vi "open motors.vi"() -> ()   [LabVIEW 2019]
uses:
  <vilib>/Rock Robotics/WPI/ThirdParty/Phoenix-LabVIEW/Motor Controller/Controls/CTRE_Phoenix_MotorControl_TalonFXMotorControllerConfigurables.ctl
  <vilib>/Rock Robotics/WPI/ThirdParty/Phoenix-LabVIEW/Motor Controller/Controls/CTRE_Phoenix_MotorControl_BaseConfigurables.ctl
  <vilib>/Rock Robotics/WPI/ThirdParty/Phoenix-LabVIEW/Motor Controller/Controls/CTRE_Phoenix_MotorControl_VelocityMeasurementPeriod.ctl
  <vilib>/Rock Robotics/WPI/ThirdParty/Phoenix-LabVIEW/Motor Controller/Controls/CTRE_Phoenix_MotorControl_SlotStructure.ctl
  <vilib>/Rock Robotics/WPI/ThirdParty/Phoenix-LabVIEW/Motor Controller/Controls/CTRE_Phoenix_MotorControl_FilterStruct.ctl
  <vilib>/Rock Robotics/WPI/ThirdParty/Phoenix-LabVIEW/Motor Controller/Controls/CTRE_Phoenix_MotorControl_RemoteSourceType.ctl
  <vilib>/Rock Robotics/WPI/ThirdParty/Phoenix-LabVIEW/Controls/CTRE_Phoenix_CustomParamConfiguration.ctl
  <vilib>/Rock Robotics/WPI/ThirdParty/Phoenix-LabVIEW/Motor Controller/Controls/CTRE_Phoenix_MotorControl_FeedbackDevice_TalonFX.ctl
  <vilib>/Rock Robotics/WPI/ThirdParty/Phoenix-LabVIEW/Motor Controller/Controls/CTRE_Phoenix_MotorControl_LimitSwitchNormal.ctl
  <vilib>/Rock Robotics/WPI/ThirdParty/Phoenix-LabVIEW/Motor Controller/Controls/CTRE_Phoenix_MotorControl_LimitSwitchSource_Local.ctl
  <vilib>/Rock Robotics/WPI/ThirdParty/Phoenix-LabVIEW/Motor Controller/Controls/CTRE_Phoenix_MotorControl_SupplyCurrentLimitConfiguration.ctl
  <vilib>/Rock Robotics/WPI/ThirdParty/Phoenix-LabVIEW/Motor Controller/Controls/CTRE_Phoenix_MotorControl_StatorCurrentLimitConfiguration.ctl
  <vilib>/Rock Robotics/WPI/ThirdParty/Phoenix-LabVIEW/Motor Controller/Controls/CTRE_Phoenix_MotorControl_MotorCommutation_TalonFX.ctl
  <vilib>/Rock Robotics/WPI/ThirdParty/Phoenix-LabVIEW/CANCoder/Controls/CTRE_Phoenix_CANcoder_AbsoluteSensorRange.ctl
  <vilib>/Rock Robotics/WPI/ThirdParty/Phoenix-LabVIEW/CANCoder/Controls/CTRE_Phoenix_CANcoder_SensorInitializationStrategy.ctl
  <vilib>/Rock Robotics/WPI/ThirdParty/Phoenix-LabVIEW/Motor Controller/Controls/CTRE_Phoenix_MotorControl_StatusFrameEnhanced.ctl
  <vilib>/Rock Robotics/WPI/ThirdParty/Phoenix-LabVIEW/Motor Controller/Controls/CTRE_Phoenix_MotorControl_EnhancedMotorControllerConfigurables.ctl
  <vilib>/Rock Robotics/WPI/ThirdParty/Phoenix-LabVIEW/Motor Controller/Controls/CTRE_Phoenix_MotorControl_FeedbackDevice.ctl
  <vilib>/Rock Robotics/WPI/ThirdParty/Phoenix-LabVIEW/Motor Controller/Controls/CTRE_Phoenix_MotorControl_SensorTermFeedbackDevice_Enhanced.ctl
  <vilib>/Rock Robotics/WPI/RobotDrive/WPI_RobotDriveOpen4MotorWithExistingMotors.vi
panel:
  in  "Talon FX Configurables":T1={"Base Configurables"={"openLoopRamp"=0.0, "closedLoopRamp"=0.0, "peakOutputForward"=1.0, "peakOutputReverse"=-1.0, "nominalOutputForward"=0.0, "nominalOutputReverse"=0.0, "neutralDeadband"=0.04, "voltageCompSaturation"=0.0, "voltageMeasurementFilter"=32, "velocityMeasurementPeriod"=100, "velocityMeasurementWindow"=64, "forwardSoftLimitThreshold"=0, "reverseSoftLimitThreshold"=0, "forwardSoftLimitEnable"=FALSE, "reverseSoftLimitEnable"=FALSE, "slot0"={"P"=0.0, "I"=0.0, "D"=0.0, "F"=0.0, "integralZone"=0.0, "allowableClosedLoopError"=0, "maxIntegralAccumulator"=0.0, "closedLoopPeakOutput"=1.0, "closedLoopPeriod"=1}, "slot1"={"P"=0.0, "I"=0.0, "D"=0.0, "F"=0.0, "integralZone"=0.0, "allowableClosedLoopError"=0, "maxIntegralAccumulator"=0.0, "closedLoopPeakOutput"=1.0, "closedLoopPeriod"=1}, "slot2"={"P"=0.0, "I"=0.0, "D"=0.0, "F"=0.0, "integralZone"=0.0, "allowableClosedLoopError"=0, "maxIntegralAccumulator"=0.0, "closedLoopPeakOutput"=1.0, "closedLoopPeriod"=1}, "slot3"={"P"=0.0, "I"=0.0, "D"=0.0, "F"=0.0, "integralZone"=0.0, "allowableClosedLoopError"=0, "maxIntegralAccumulator"=0.0, "closedLoopPeakOutput"=1.0, "closedLoopPeriod"=1}, "auxPIDPolarity"=FALSE, "remoteFilter0"={"remoteSensorDeviceID"=0, "remoteSensorSource"=enum."Off"}, "remoteFilter1"={"remoteSensorDeviceID"=0, "remoteSensorSource"=enum."Off"}, "motionCruiseVelocity"=0, "motionAcceleration"=0, "motionProfileTrajectoryPeriod"=0, "feedbackNotContinuous"=FALSE, "remoteSensorClosedLoopDisableNeutralOnLOS"=FALSE, "clearPositionOnLimitF"=FALSE, "clearPositionOnLimitR"=FALSE, "clearPositionOnQuadIdx"=FALSE, "limitSwitchDisableNeutralOnLOS"=FALSE, "softLimitDisableNeutralOnLOS"=FALSE, "pulseWidthPeriod_EdgesPerRot"=1, "pulseWidthPeriod_FilterWindowSz"=1, "customParam"={"customParam0"=0, "customParam1"=0}, "trajectoryInterpolationEnable"=TRUE}, "primaryPID"={"selectedFeedbackCoefficient"=1.0, "selectedFeedbackSensor"=1}, "auxiliaryPID"={"selectedFeedbackCoefficient"=1.0, "selectedFeedbackSensor"=1}, "forwardLimitSwitchNormal"=enum."Normally Open", "reverseLimitSwitchNormal"=enum."Normally Open", "forwardLimitSwitchDeviceID"=0, "reverseLimitSwitchDeviceID"=0, "forwardLimitSwitchSource"=enum."Feedback Connector", "reverseLimitSwitchSource"=enum."Feedback Connector", "sum0Term"=1, "sum1Term"=1, "diff0Term"=1, "diff1Term"=1, "Supply Current Limit Configuration"={"Enable?"=FALSE, "Current Limit"=0.0, "Threshold Current"=0.0, "Threshold Time"=0.0}, "Stator Current Limit Configuration"={"Enable?"=FALSE, "Current Limit"=0.0, "Threshold Current"=0.0, "Threshold Time"=0.0}, "Motor Commutation"=enum."Trapezoidal", "Absolute Sensor Range"=enum."Unsigned [0 to 360)", "Integrated Sensor Offset (Degrees)"=0.0, "Sensor Initialization Strategy"=enum."Boot To Zero"} {"diff1Term" items=["Integrated Sensor"=1, "Sensor Sum (S0 + S1)"=9, "Sensor Difference (D0 - D1)"=10, "Remote Source 0"=11, "Remote Source 1"=12, "None"=14, "Software Emulated"=15]; "diff0Term" items=["Integrated Sensor"=1, "Sensor Sum (S0 + S1)"=9, "Sensor Difference (D0 - D1)"=10, "Remote Source 0"=11, "Remote Source 1"=12, "None"=14, "Software Emulated"=15]; "sum1Term" items=["Integrated Sensor"=1, "Sensor Sum (S0 + S1)"=9, "Sensor Difference (D0 - D1)"=10, "Remote Source 0"=11, "Remote Source 1"=12, "None"=14, "Software Emulated"=15]; "sum0Term" items=["Integrated Sensor"=1, "Sensor Sum (S0 + S1)"=9, "Sensor Difference (D0 - D1)"=10, "Remote Source 0"=11, "Remote Source 1"=12, "None"=14, "Software Emulated"=15]; "auxiliaryPID"."selectedFeedbackSensor" items=["Integrated Sensor"=1, "Sensor Sum (S0 + S1)"=9, "Sensor Difference (D0 - D1)"=10, "Remote Source 0"=11, "Remote Source 1"=12, "None"=14, "Software Emulated"=15]; "primaryPID"."selectedFeedbackSensor" items=["Integrated Sensor"=1, "Sensor Sum (S0 + S1)"=9, "Sensor Difference (D0 - D1)"=10, "Remote Source 0"=11, "Remote Source 1"=12, "None"=14, "Software Emulated"=15]; "Base Configurables"."velocityMeasurementPeriod" items=["Period_1ms"=1, "Period_2ms"=2, "Period_5ms"=5, "Period_10ms"=10, "Period_20ms"=20, "Period_25ms"=25, "Period_50ms"=50, "Period_100ms"=100]}
  in  "Tune PIDF Manually?":bool
  in  "Back Motor PIDF Values":cluster{"P":dbl, "I":dbl, "D":dbl, "F":dbl}
  in  "Front Motor PIDF Values":cluster{"P":dbl, "I":dbl, "D":dbl, "F":dbl}
  in  "Tune PIDF Manually? 2":bool
  in  "Back Motor PIDF Values 2":cluster{"P":dbl, "I":dbl, "D":dbl, "F":dbl}
  in  "Front Motor PIDF Values 2":cluster{"P":dbl, "I":dbl, "D":dbl, "F":dbl}
  # "After you have the gains you want,\nRight-Click > Data Operations > Make the Current Value Default"
  # "Sum and Diff terms are ways to select more than one sensor as a feedback device. \n Sum 0 is the first feedback device to be used for the Sum term.\n Sum 1 is the feedback device to be added to Sum 0 for the Sum term.\n Diff 0 and Diff 1 work in a similar manner."
  # "These are only applicable\nif using a remote limit switch.\n\nLocal limit switches/no limit\nswitches do not use this."
  # "Current is below Current Limit AND\n\n(Requested output is weaker** than applied motor\noutput OR is in the opposite direction).\n/\nMotor output is set to requested output."
  # "Current is above Threshold Current for Threshold Time\n/\nReduce motor output (towards neutral)."
  # "Current is below Current Limit.\n/\nRamp motor output towards requested output."
  # "Current is above Current Limit.\n/\nReduce motor output (towards neutral)."
  # "*If the configured Peak Threshold is less than the Continuous Threshold, the applied Peak Threshold is set equal to the Configured Continuous Threshold in firmware.\n** Both requested output and applied motor output are in the same direction, and requested output is closer to neutral."
  # "False: Primary Output = PID[0] + PID[1]  ---  Auxiliary Output = PID[0] - PID[1]\nTrue:  Primary Output = PID[0] - PID[1] --- Auxiliary Output = PID[0] + PID[1]"
  # "Enable the motion profile executor to perform linear interpolation between profile points.  Defaults to True."
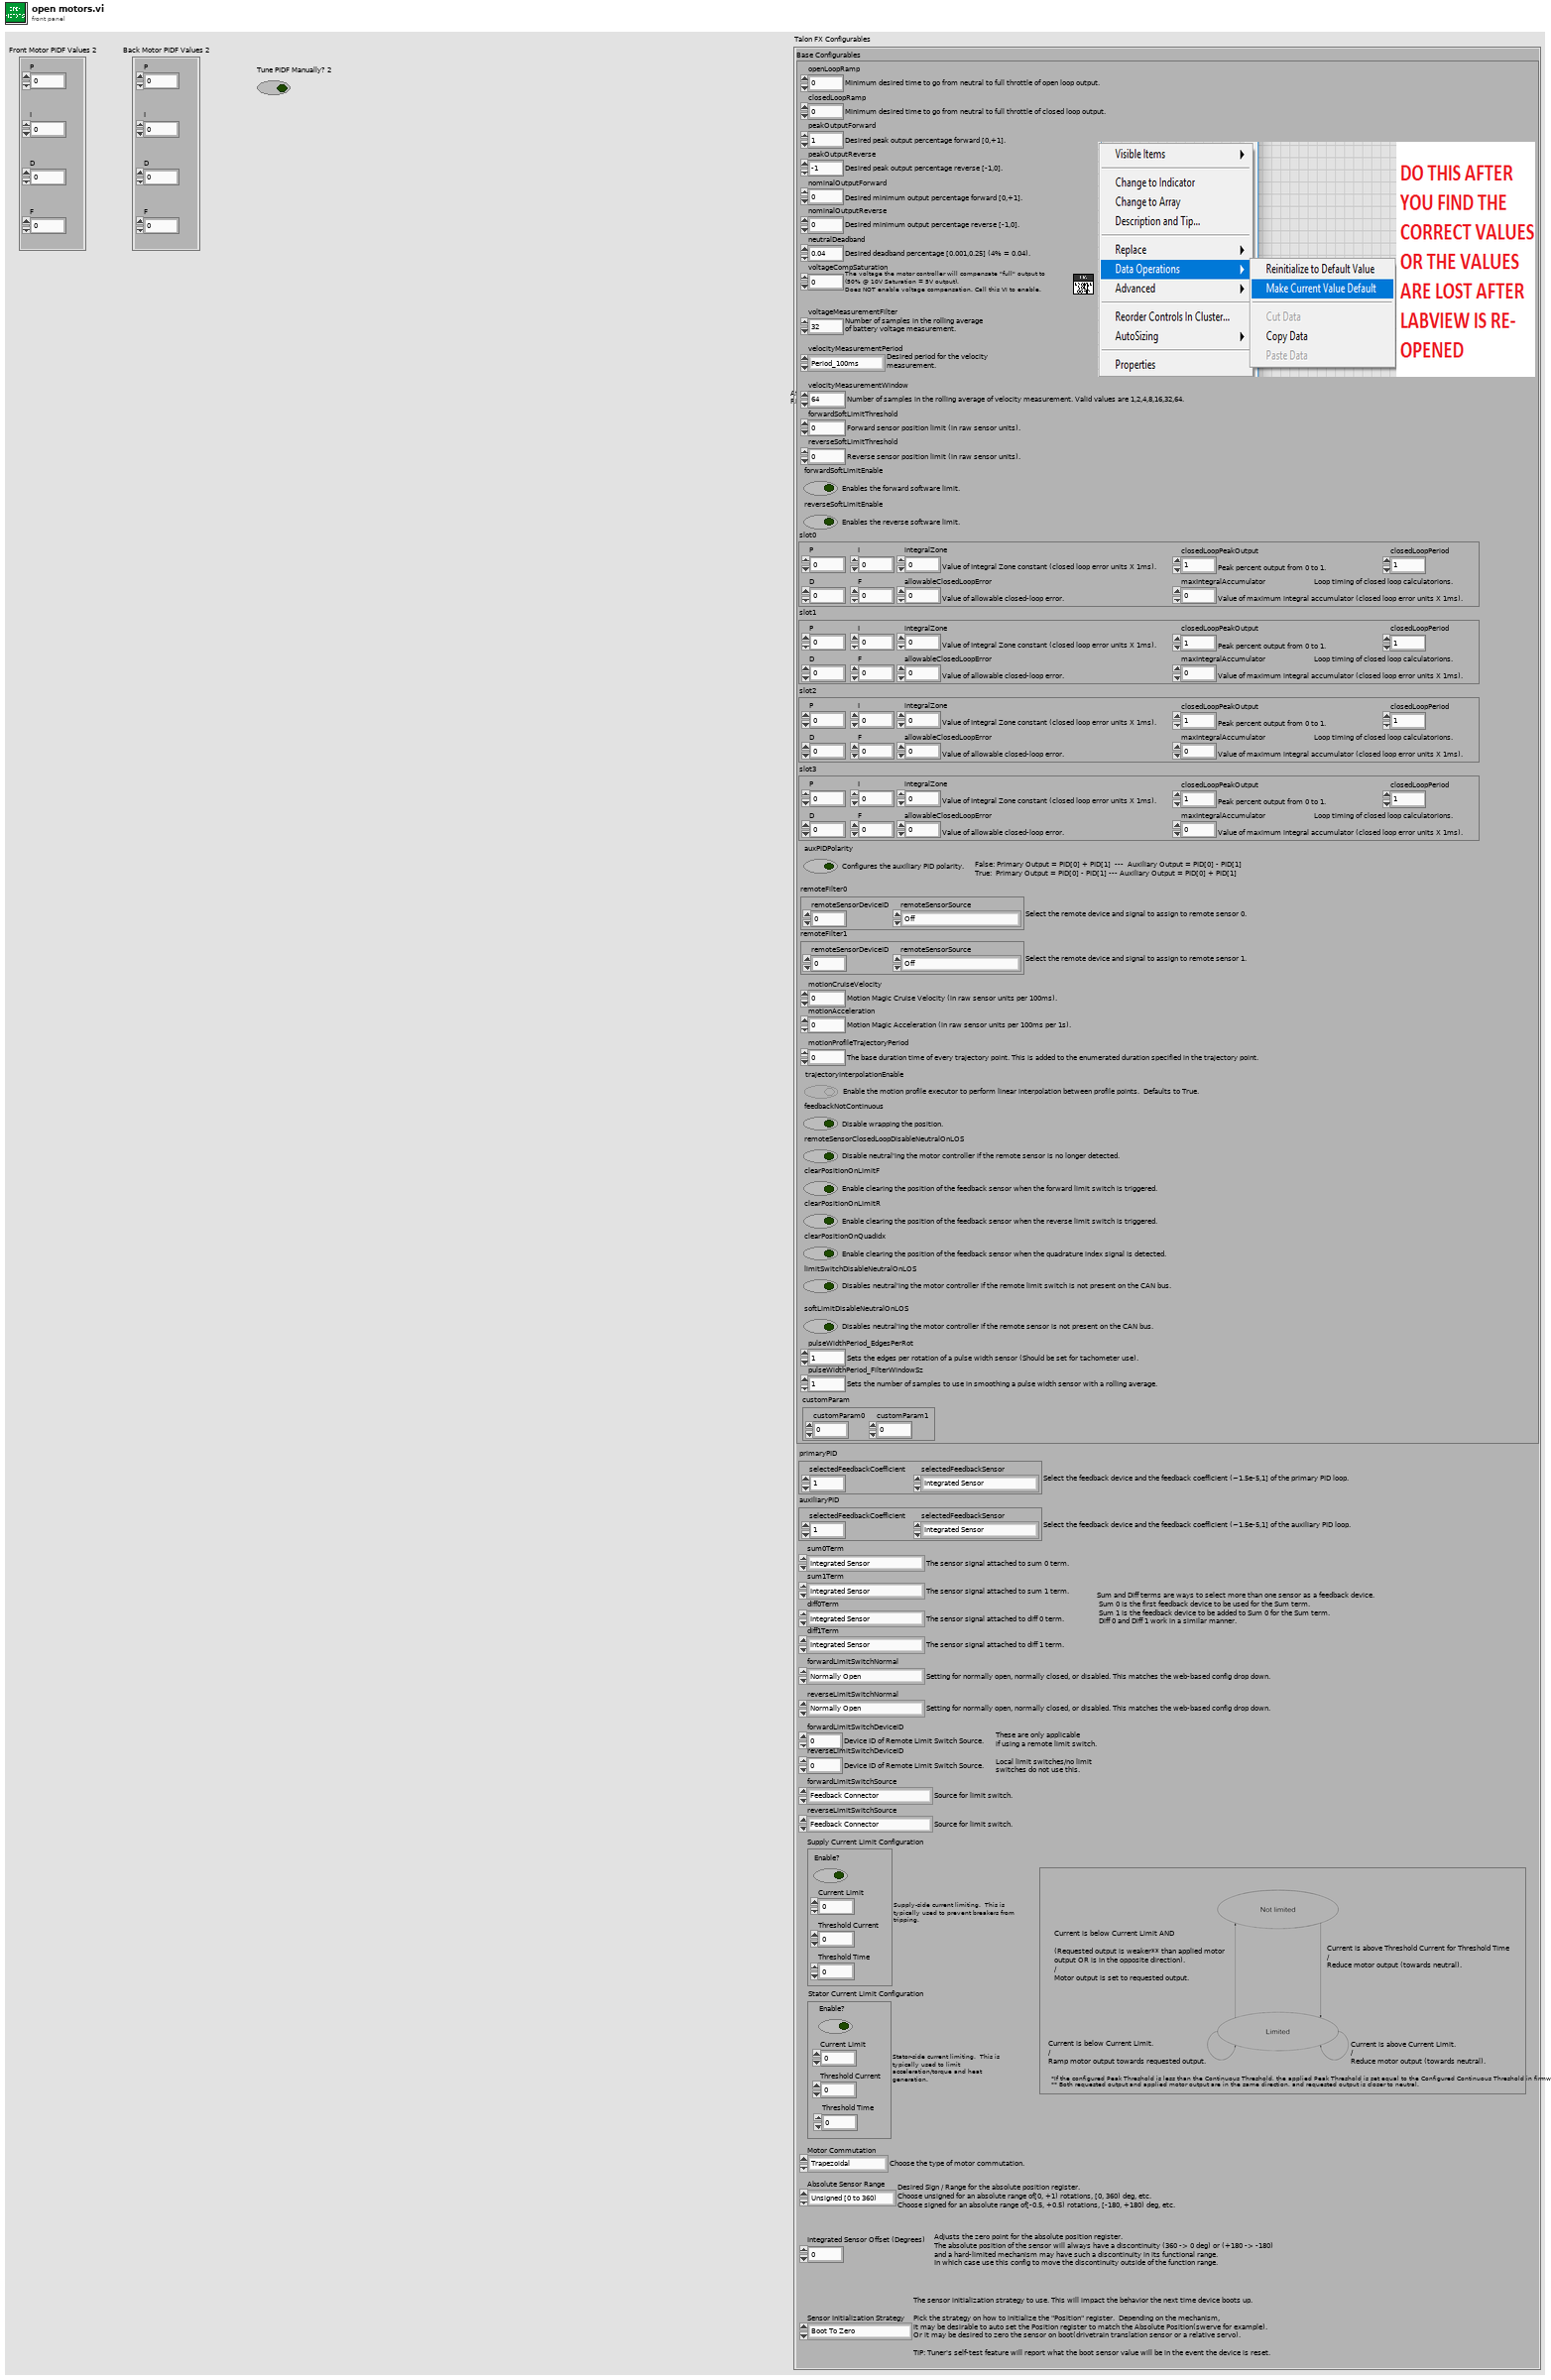
[diagram p1: front panel]
types:
  T1 = typedef "CTRE_Phoenix_MotorControl_TalonFXMotorControllerConfigurables.ctl" = cluster{"Base Configurables":T2, "primaryPID":cluster{"selectedFeedbackCoefficient":dbl, "selectedFeedbackSensor":T8}, "auxiliaryPID":cluster{"selectedFeedbackCoefficient":dbl, "selectedFeedbackSensor":T8}, "forwardLimitSwitchNormal":T9, "reverseLimitSwitchNormal":T9, "forwardLimitSwitchDeviceID":i32, "reverseLimitSwitchDeviceID":i32, "forwardLimitSwitchSource":T10, "reverseLimitSwitchSource":T10, "sum0Term":T8, "sum1Term":T8, "diff0Term":T8, "diff1Term":T8, "Supply Current Limit Configuration":T11, "Stator Current Limit Configuration":T12, "Motor Commutation":T13, "Absolute Sensor Range":T14, "Integrated Sensor Offset (Degrees)":dbl, "Sensor Initialization Strategy":T15}
  T2 = typedef "CTRE_Phoenix_MotorControl_BaseConfigurables.ctl" = cluster{"openLoopRamp":dbl, "closedLoopRamp":dbl, "peakOutputForward":dbl, "peakOutputReverse":dbl, "nominalOutputForward":dbl, "nominalOutputReverse":dbl, "neutralDeadband":dbl, "voltageCompSaturation":dbl, "voltageMeasurementFilter":i32, "velocityMeasurementPeriod":T3, "velocityMeasurementWindow":i32, "forwardSoftLimitThreshold":i32, "reverseSoftLimitThreshold":i32, "forwardSoftLimitEnable":bool, "reverseSoftLimitEnable":bool, "slot0":T4, "slot1":T4, "slot2":T4, "slot3":T4, "auxPIDPolarity":bool, "remoteFilter0":T5, "remoteFilter1":T5, "motionCruiseVelocity":i32, "motionAcceleration":i32, "motionProfileTrajectoryPeriod":i32, "feedbackNotContinuous":bool, "remoteSensorClosedLoopDisableNeutralOnLOS":bool, "clearPositionOnLimitF":bool, "clearPositionOnLimitR":bool, "clearPositionOnQuadIdx":bool, "limitSwitchDisableNeutralOnLOS":bool, "softLimitDisableNeutralOnLOS":bool, "pulseWidthPeriod_EdgesPerRot":i32, "pulseWidthPeriod_FilterWindowSz":i32, "customParam":T7, "trajectoryInterpolationEnable":bool}
  T3 = typedef "CTRE_Phoenix_MotorControl_VelocityMeasurementPeriod.ctl" = u16
  T4 = typedef "CTRE_Phoenix_MotorControl_SlotStructure.ctl" = cluster{"P":dbl, "I":dbl, "D":dbl, "F":dbl, "integralZone":dbl, "allowableClosedLoopError":i32, "maxIntegralAccumulator":dbl, "closedLoopPeakOutput":dbl, "closedLoopPeriod":i32}
  T5 = typedef "CTRE_Phoenix_MotorControl_FilterStruct.ctl" = cluster{"remoteSensorDeviceID":u8, "remoteSensorSource":T6}
  T6 = typedef "CTRE_Phoenix_MotorControl_RemoteSourceType.ctl" = enum16{"Off", "Talon SRX Selected Sensor", "Pigeon IMU Yaw", "Pigeon IMU Pitch", "Pigeon IMU Roll", "CANifier Quadrature", "CANifier PWM Input 0", "CANifier PWM Input 1", "CANifier PWM Input 2", "CANifier PWM Input 3", "Gadgeteer Pigeon Yaw", "Gadgeteer Pigeon Pitch", "Gadgeteer Pigeon Roll"}
  T7 = typedef "CTRE_Phoenix_CustomParamConfiguration.ctl" = cluster{"customParam0":i32, "customParam1":i32}
  T8 = typedef "CTRE_Phoenix_MotorControl_FeedbackDevice_TalonFX.ctl" = i8
  T9 = typedef "CTRE_Phoenix_MotorControl_LimitSwitchNormal.ctl" = enum16{"Normally Open", "Normally Closed", "Disabled"}
  T10 = typedef "CTRE_Phoenix_MotorControl_LimitSwitchSource_Local.ctl" = enum16{"Feedback Connector", "Remote Talon SRX", "Remote CANifier", "Deactivated"}
  T11 = typedef "CTRE_Phoenix_MotorControl_SupplyCurrentLimitConfiguration.ctl" = cluster{"Enable?":bool, "Current Limit":dbl, "Threshold Current":dbl, "Threshold Time":dbl}
  T12 = typedef "CTRE_Phoenix_MotorControl_StatorCurrentLimitConfiguration.ctl" = cluster{"Enable?":bool, "Current Limit":dbl, "Threshold Current":dbl, "Threshold Time":dbl}
  T13 = typedef "CTRE_Phoenix_MotorControl_MotorCommutation_TalonFX.ctl" = enum16{"Trapezoidal"}
  T14 = typedef "CTRE_Phoenix_CANcoder_AbsoluteSensorRange.ctl" = enum16{"Unsigned [0 to 360)", "Signed [-180 to +180)"}
  T15 = typedef "CTRE_Phoenix_CANcoder_SensorInitializationStrategy.ctl" = enum16{"Boot To Zero", "Boot To Absolute Position"}
  T16 = typedef "CTRE_Phoenix_MotorControl_EnhancedMotorControllerConfigurables.ctl" = cluster{"Base Configurables":T2, "primaryPID":cluster{"selectedFeedbackCoefficient":dbl, "selectedFeedbackSensor":T17}, "auxiliaryPID":cluster{"selectedFeedbackCoefficient":dbl, "selectedFeedbackSensor":T17}, "sum0Term":T18, "sum1Term":T18, "diff0Term":T18, "diff1Term":T18, "forwardLimitSwitchNormal":T9, "reverseLimitSwitchNormal":T9, "forwardLimitSwitchDeviceID":i32, "reverseLimitSwitchDeviceID":i32, "forwardLimitSwitchSource":T10, "reverseLimitSwitchSource":T10, "peakCurrentLimit":i32, "peakCurrentDuration":i32, "continuousCurrentLimit":i32}
  T17 = typedef "CTRE_Phoenix_MotorControl_FeedbackDevice.ctl" = i8
  T18 = typedef "CTRE_Phoenix_MotorControl_SensorTermFeedbackDevice_Enhanced.ctl" = i8
  T19 = typedef "CTRE_Phoenix_MotorControl_StatusFrameEnhanced.ctl" = u16
  T20 = typedef "WPI_MotorControlDeviceRef.ctl" = cluster{"DeviceStatus":errorcluster, "Type":T21, "PWM":cluster{"PWM Channel":T22, "DeadBand":T23}, "CAN":cluster{"Device Number":u8, "SetOutput VI Ref":variant, "GetOutput VI Ref":variant, "Enable VI Ref":variant, "Disable VI Ref":variant, "Data":variant}, "Invert":bool, "DIO PWM":cluster{"PWM \"Enable\" Channel":T22, "DIOChannel":T24, "PWM Rate":dbl}}
  T21 = typedef "WPI_MotorControlType.ctl" = enum16{"PWM", "CAN", "DIO PWM"}
  T22 = typedef "FPGA_DIOPWMChannel.ctl" = enum8{"PWM 0", "PWM 1", "PWM 2", "PWM 3", "PWM 4", "PWM 5", "PWM 6", "PWM 7", "PWM 8", "PWM 9", "PWM MXP 0", "PWM MXP 1", "PWM MXP 2", "PWM MXP 3", "PWM MXP 4", "PWM MXP 5", "PWM MXP 6", "PWM MXP 7", "PWM MXP 8", "PWM MXP 9", "Invalid"}
  T23 = typedef "WPI_PWMDeadband.ctl" = cluster{"Name":string, "maxPositivePwm":i32, "minPositivePwm":i32, "centerPwm":i32, "maxNegativePwm":i32, "minNegativePwm":i32, "angularRange":u16}
  T24 = typedef "FPGA_DIOChannel.ctl" = enum8{"DIO 0", "DIO 1", "DIO 2", "DIO 3", "DIO 4", "DIO 5", "DIO 6", "DIO 7", "DIO 8", "DIO 9", "DIO MXP 0", "DIO MXP 1", "DIO MXP 2", "DIO MXP 3", "DIO MXP 4", "DIO MXP 5", "DIO MXP 6", "DIO MXP 7", "DIO MXP 8", "DIO MXP 9", "DIO MXP 10", "DIO MXP 11", "DIO MXP 12", "DIO MXP 13", "DIO MXP 14", "DIO MXP 15", "SPI Port CS1", "SPI Port CS2", "SPI Port CS3", "SPI Port MISO", "SPI Port MOSI", "Invalid"}
  T25 = typedef "WPI_RobotDriveDevRef.ctl" = cluster{"DevStatus":errorcluster, "Motors[]":T20[], "Square Inputs":bool, "Max Output":dbl}
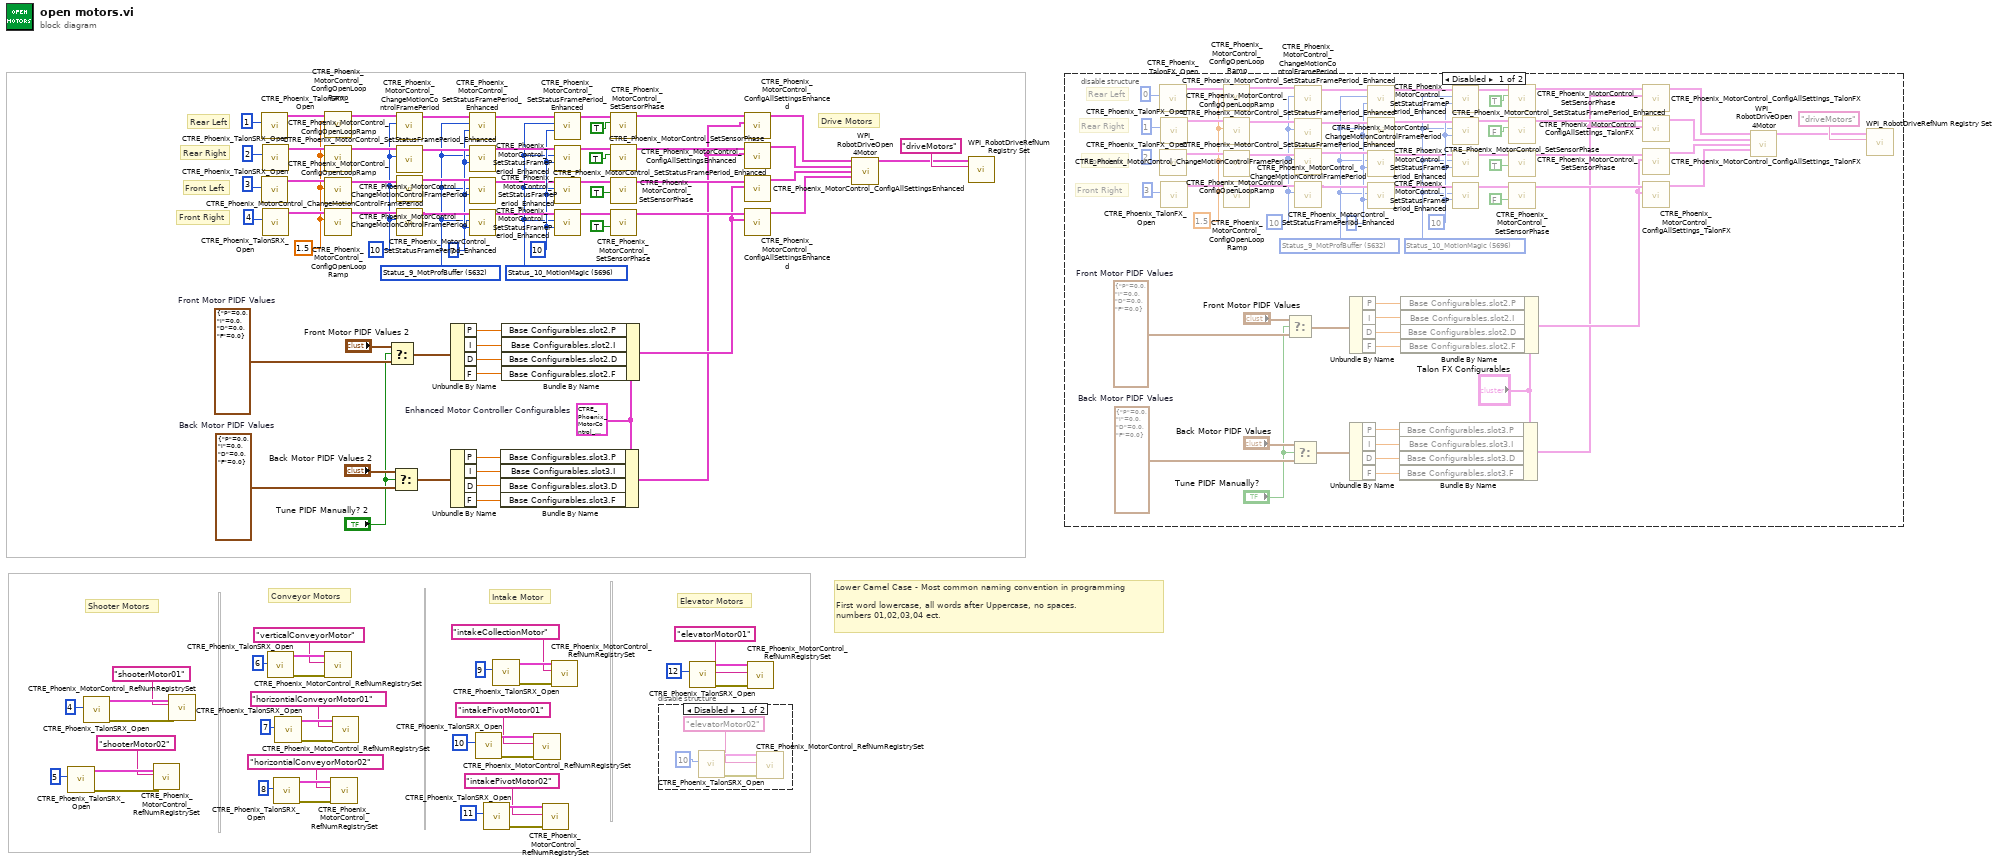
[diagram p0: block diagram]
diagram:
  w19 = T16 {"Base Configurables"={"openLoopRamp"=0.0, "closedLoopRamp"=0.0, "peakOutputForward"=1.0, "peakOutputReverse"=-1.0, "nominalOutputForward"=0.0, "nominalOutputReverse"=0.0, "neutralDeadband"=0.04, "voltageCompSaturation"=0.0, "voltageMeasurementFilter"=32, "velocityMeasurementPeriod"=100, "velocityMeasurementWindow"=64, "forwardSoftLimitThreshold"=0, "reverseSoftLimitThreshold"=0, "forwardSoftLimitEnable"=FALSE, "reverseSoftLimitEnable"=FALSE, "slot0"={"P"=0.0, "I"=0.0, "D"=0.0, "F"=0.0, "integralZone"=0.0, "allowableClosedLoopError"=0, "maxIntegralAccumulator"=0.0, "closedLoopPeakOutput"=1.0, "closedLoopPeriod"=1}, "slot1"={"P"=0.0, "I"=0.0, "D"=0.0, "F"=0.0, "integralZone"=0.0, "allowableClosedLoopError"=0, "maxIntegralAccumulator"=0.0, "closedLoopPeakOutput"=1.0, "closedLoopPeriod"=1}, "slot2"={"P"=0.0, "I"=0.0, "D"=0.0, "F"=0.0, "integralZone"=0.0, "allowableClosedLoopError"=0, "maxIntegralAccumulator"=0.0, "closedLoopPeakOutput"=1.0, "closedLoopPeriod"=1}, "slot3"={"P"=0.0, "I"=0.0, "D"=0.0, "F"=0.0, "integralZone"=0.0, "allowableClosedLoopError"=0, "maxIntegralAccumulator"=0.0, "closedLoopPeakOutput"=1.0, "closedLoopPeriod"=1}, "auxPIDPolarity"=FALSE, "remoteFilter0"={"remoteSensorDeviceID"=0, "remoteSensorSource"=enum."Off"}, "remoteFilter1"={"remoteSensorDeviceID"=0, "remoteSensorSource"=enum."Off"}, "motionCruiseVelocity"=0, "motionAcceleration"=0, "motionProfileTrajectoryPeriod"=0, "feedbackNotContinuous"=FALSE, "remoteSensorClosedLoopDisableNeutralOnLOS"=FALSE, "clearPositionOnLimitF"=FALSE, "clearPositionOnLimitR"=FALSE, "clearPositionOnQuadIdx"=FALSE, "limitSwitchDisableNeutralOnLOS"=FALSE, "softLimitDisableNeutralOnLOS"=FALSE, "pulseWidthPeriod_EdgesPerRot"=1, "pulseWidthPeriod_FilterWindowSz"=1, "customParam"={"customParam0"=0, "customParam1"=0}, "trajectoryInterpolationEnable"=TRUE}, "primaryPID"={"selectedFeedbackCoefficient"=1.0, "selectedFeedbackSensor"=0}, "auxiliaryPID"={"selectedFeedbackCoefficient"=1.0, "selectedFeedbackSensor"=0}, "sum0Term"=0, "sum1Term"=0, "diff0Term"=0, "diff1Term"=0, "forwardLimitSwitchNormal"=enum."Normally Open", "reverseLimitSwitchNormal"=enum."Normally Open", "forwardLimitSwitchDeviceID"=0, "reverseLimitSwitchDeviceID"=0, "forwardLimitSwitchSource"=enum."Feedback Connector", "reverseLimitSwitchSource"=enum."Feedback Connector", "peakCurrentLimit"=1, "peakCurrentDuration"=1, "continuousCurrentLimit"=1}  # Enhanced Motor Controller Configurables
  w33 = cluster{"P":dbl, "I":dbl, "D":dbl, "F":dbl} {"P"=0.0, "I"=0.0, "D"=0.0, "F"=0.0}  # Back Motor PIDF Values
  w34 = cluster{"P":dbl, "I":dbl, "D":dbl, "F":dbl} {"P"=0.0, "I"=0.0, "D"=0.0, "F"=0.0}  # Front Motor PIDF Values
  w51 = T19 5696 items=["Status_1_General"=5120, "Status_2_Feedback0"=5184, "Status_3_Quadrature"=5248, "Status_4_AinTempVbat"=5312, "Status_6_Misc"=5440, "Status_7_CommStatus"=5504, "Status_8_PulseWidth"=5568, "Status_9_MotProfBuffer"=5632, "Status_10_MotionMagic"=5696, "Status_11_UartGadgeteer"=5760, "Status_12_Feedback1"=5824, "Status_13_Base_PIDF0"=5888, "Status_14_Turn_PIDF1"=5952, "Status_15_FirmwareApiStatus"=6016] ("Status Frame")
  w53 = T19 5632 items=["Status_1_General"=5120, "Status_2_Feedback0"=5184, "Status_3_Quadrature"=5248, "Status_4_AinTempVbat"=5312, "Status_6_Misc"=5440, "Status_7_CommStatus"=5504, "Status_8_PulseWidth"=5568, "Status_9_MotProfBuffer"=5632, "Status_10_MotionMagic"=5696, "Status_11_UartGadgeteer"=5760, "Status_12_Feedback1"=5824, "Status_13_Base_PIDF0"=5888, "Status_14_Turn_PIDF1"=5952, "Status_15_FirmwareApiStatus"=6016] ("Status Frame")
  w55 = 7
  w54 = 10
  w63 = 10
  w68 = 1.5
  # "Front Right"
  # "Front Left"
  # "Rear Right"
  # "Rear Left"
  # "Drive Motors"
  # "Lower Camel Case - Most common naming convention in programming\n\nFirst word lowercase, all words after Uppercase, no spaces.\nnumbers 01,02,03,04 ect."
  # "Elevator Motors"
  # "Intake Motor"
  # "Conveyor Motors"
  # "Shooter Motors"
  n1 = call <vilib>:"CTRE_Phoenix_TalonSRX_Open.vi"("Device Number"=u8 5) -> ("error out"=w15:errorcluster, "CAN Talon SRX Ref"=w14:T20)  [unwired: 9 in]
  n2 = call <vilib>:"CTRE_Phoenix_TalonSRX_Open.vi"("Device Number"=u8 4) -> ("error out"=w97:errorcluster, "CAN Talon SRX Ref"=w96:T20)  [unwired: 9 in]
  n3 = call <vilib>:"CTRE_Phoenix_MotorControl_RefNumRegistrySet.vi"("error in (no error)"=w15, "refnum name"="shooterMotor02", "PhoenixMotorControlDevRef"=w14) -> ()  [unwired: 7 in, 2 out]
  n4 = call <vilib>:"CTRE_Phoenix_MotorControl_RefNumRegistrySet.vi"("error in (no error)"=w97, "refnum name"="shooterMotor01", "PhoenixMotorControlDevRef"=w96) -> ()  [unwired: 7 in, 2 out]
  n5 = call <vilib>:"CTRE_Phoenix_TalonSRX_Open.vi"("Device Number"=u8 1) -> ("CAN Talon SRX Ref"=w72:T20)  [unwired: 9 in, 1 out]
  n6 = call <vilib>:"CTRE_Phoenix_TalonSRX_Open.vi"("Device Number"=u8 3) -> ("CAN Talon SRX Ref"=w70:T20)  [unwired: 9 in, 1 out]
  n7 = call <vilib>:"CTRE_Phoenix_TalonSRX_Open.vi"("Device Number"=u8 2) -> ("CAN Talon SRX Ref"=w71:T20)  [unwired: 9 in, 1 out]
  n8 = call <vilib>:"CTRE_Phoenix_TalonSRX_Open.vi"("Device Number"=u8 4) -> ("CAN Talon SRX Ref"=w69:T20)  [unwired: 9 in, 1 out]
  n9 = call <vilib>:"CTRE_Phoenix_TalonSRX_Open.vi"("Device Number"=u8 6) -> ("error out"=w92:errorcluster, "CAN Talon SRX Ref"=w93:T20)  [unwired: 9 in]
  n10 = call <vilib>:"CTRE_Phoenix_TalonSRX_Open.vi"("Device Number"=u8 8) -> ("error out"=w6:errorcluster, "CAN Talon SRX Ref"=w7:T20)  [unwired: 9 in]
  n11 = call <vilib>:"CTRE_Phoenix_TalonSRX_Open.vi"("Device Number"=u8 7) -> ("error out"=w10:errorcluster, "CAN Talon SRX Ref"=w11:T20)  [unwired: 9 in]
  n12 = call <vilib>:"CTRE_Phoenix_MotorControl_ConfigOpenLoopRamp.vi"("secondsFromNeutralToFull"=w68, "PhoenixMotorControlDevRef"=w72) -> ("PhoenixMotorControlDevRef"=w67:T20)  [unwired: 8 in, 1 out]
  n13 = call <vilib>:"CTRE_Phoenix_MotorControl_ConfigOpenLoopRamp.vi"("secondsFromNeutralToFull"=w68, "PhoenixMotorControlDevRef"=w71) -> ("PhoenixMotorControlDevRef"=w66:T20)  [unwired: 8 in, 1 out]
  n14 = call <vilib>:"CTRE_Phoenix_MotorControl_ConfigOpenLoopRamp.vi"("secondsFromNeutralToFull"=w68, "PhoenixMotorControlDevRef"=w70) -> ("PhoenixMotorControlDevRef"=w65:T20)  [unwired: 8 in, 1 out]
  n15 = call <vilib>:"CTRE_Phoenix_MotorControl_ConfigOpenLoopRamp.vi"("secondsFromNeutralToFull"=w68, "PhoenixMotorControlDevRef"=w69) -> ("PhoenixMotorControlDevRef"=w64:T20)  [unwired: 8 in, 1 out]
  n16 = call <vilib>:"CTRE_Phoenix_MotorControl_RefNumRegistrySet.vi"("error in (no error)"=w92, "refnum name"="verticalConveyorMotor", "PhoenixMotorControlDevRef"=w93) -> ()  [unwired: 7 in, 2 out]
  n17 = call <vilib>:"CTRE_Phoenix_MotorControl_RefNumRegistrySet.vi"("error in (no error)"=w6, "refnum name"="horizontialConveyorMotor02", "PhoenixMotorControlDevRef"=w7) -> ()  [unwired: 7 in, 2 out]
  n18 = call <vilib>:"CTRE_Phoenix_MotorControl_RefNumRegistrySet.vi"("error in (no error)"=w10, "refnum name"="horizontialConveyorMotor01", "PhoenixMotorControlDevRef"=w11) -> ()  [unwired: 7 in, 2 out]
  n19 = Select(t="Front Motor PIDF Values 2", s="Tune PIDF Manually? 2", f=w34) -> (s? t:f=w30:cluster{"P":dbl, "I":dbl, "D":dbl, "F":dbl})
  n20 = Select(t="Back Motor PIDF Values 2", s="Tune PIDF Manually? 2", f=w33) -> (s? t:f=w29:cluster{"P":dbl, "I":dbl, "D":dbl, "F":dbl})
  n21 = call <vilib>:"CTRE_Phoenix_MotorControl_ChangeMotionControlFramePeriod.vi"("periodMs"=w63, "PhoenixMotorControlDevRef"=w67) -> ("PhoenixMotorControlDevRef"=w62:T20)  [unwired: 8 in, 1 out]
  n22 = call <vilib>:"CTRE_Phoenix_MotorControl_ChangeMotionControlFramePeriod.vi"("periodMs"=w63, "PhoenixMotorControlDevRef"=w66) -> ("PhoenixMotorControlDevRef"=w61:T20)  [unwired: 8 in, 1 out]
  n23 = call <vilib>:"CTRE_Phoenix_MotorControl_ChangeMotionControlFramePeriod.vi"("periodMs"=w63, "PhoenixMotorControlDevRef"=w65) -> ("PhoenixMotorControlDevRef"=w60:T20)  [unwired: 8 in, 1 out]
  n24 = call <vilib>:"CTRE_Phoenix_MotorControl_ChangeMotionControlFramePeriod.vi"("periodMs"=w63, "PhoenixMotorControlDevRef"=w64) -> ("PhoenixMotorControlDevRef"=w59:T20)  [unwired: 8 in, 1 out]
  n25 = Unbundle By Name(w30) -> ("P"=w28:dbl, "I"=w27:dbl, "D"=w26:dbl, "F"=w25:dbl)
  n26 = Unbundle By Name(w29) -> ("P"=w24:dbl, "I"=w23:dbl, "D"=w22:dbl, "F"=w21:dbl)
  n27 = call <vilib>:"CTRE_Phoenix_MotorControl_SetStatusFramePeriod_Enhanced.vi"("periodMs"=w55, "Status Frame"=w53, "PhoenixMotorControlDevRef"=w62) -> ("PhoenixMotorControlDevRef"=w58:T20)  [unwired: 7 in, 1 out]
  n28 = call <vilib>:"CTRE_Phoenix_MotorControl_SetStatusFramePeriod_Enhanced.vi"("periodMs"=w55, "Status Frame"=w53, "PhoenixMotorControlDevRef"=w61) -> ("PhoenixMotorControlDevRef"=w57:T20)  [unwired: 7 in, 1 out]
  n29 = call <vilib>:"CTRE_Phoenix_MotorControl_SetStatusFramePeriod_Enhanced.vi"("periodMs"=w55, "Status Frame"=w53, "PhoenixMotorControlDevRef"=w60) -> ("PhoenixMotorControlDevRef"=w52:T20)  [unwired: 7 in, 1 out]
  n30 = call <vilib>:"CTRE_Phoenix_MotorControl_SetStatusFramePeriod_Enhanced.vi"("periodMs"=w55, "Status Frame"=w53, "PhoenixMotorControlDevRef"=w59) -> ("PhoenixMotorControlDevRef"=w56:T20)  [unwired: 7 in, 1 out]
  n31 = call <vilib>:"CTRE_Phoenix_TalonSRX_Open.vi"("Device Number"=u8 10) -> ("error out"=w81:errorcluster, "CAN Talon SRX Ref"=w82:T20)  [unwired: 9 in]
  n32 = call <vilib>:"CTRE_Phoenix_TalonSRX_Open.vi"("Device Number"=u8 11) -> ("error out"=w3:errorcluster, "CAN Talon SRX Ref"=w4:T20)  [unwired: 9 in]
  n33 = call <vilib>:"CTRE_Phoenix_TalonSRX_Open.vi"("Device Number"=u8 9) -> ("error out"=w89:errorcluster, "CAN Talon SRX Ref"=w90:T20)  [unwired: 9 in]
  n34 = Bundle By Name(cluster=w19, "Base Configurables.slot3.P"=w24, "Base Configurables.slot3.I"=w23, "Base Configurables.slot3.D"=w22, "Base Configurables.slot3.F"=w21) -> (w17:T16)
  n35 = Bundle By Name(cluster=w19, "Base Configurables.slot2.P"=w28, "Base Configurables.slot2.I"=w27, "Base Configurables.slot2.D"=w26, "Base Configurables.slot2.F"=w25) -> (w18:T16)
  n36 = call <vilib>:"CTRE_Phoenix_MotorControl_RefNumRegistrySet.vi"("error in (no error)"=w81, "refnum name"="intakePivotMotor01", "PhoenixMotorControlDevRef"=w82) -> ()  [unwired: 7 in, 2 out]
  n37 = call <vilib>:"CTRE_Phoenix_MotorControl_RefNumRegistrySet.vi"("error in (no error)"=w3, "refnum name"="intakePivotMotor02", "PhoenixMotorControlDevRef"=w4) -> ()  [unwired: 7 in, 2 out]
  n38 = call <vilib>:"CTRE_Phoenix_MotorControl_RefNumRegistrySet.vi"("error in (no error)"=w89, "refnum name"="intakeCollectionMotor", "PhoenixMotorControlDevRef"=w90) -> ()  [unwired: 7 in, 2 out]
  n39 = call <vilib>:"CTRE_Phoenix_MotorControl_SetStatusFramePeriod_Enhanced.vi"("periodMs"=w54, "Status Frame"=w51, "PhoenixMotorControlDevRef"=w58) -> ("PhoenixMotorControlDevRef"=w50:T20)  [unwired: 7 in, 1 out]
  n40 = call <vilib>:"CTRE_Phoenix_MotorControl_SetStatusFramePeriod_Enhanced.vi"("periodMs"=w54, "Status Frame"=w51, "PhoenixMotorControlDevRef"=w57) -> ("PhoenixMotorControlDevRef"=w49:T20)  [unwired: 7 in, 1 out]
  n41 = call <vilib>:"CTRE_Phoenix_MotorControl_SetStatusFramePeriod_Enhanced.vi"("periodMs"=w54, "Status Frame"=w51, "PhoenixMotorControlDevRef"=w52) -> ("PhoenixMotorControlDevRef"=w48:T20)  [unwired: 7 in, 1 out]
  n42 = call <vilib>:"CTRE_Phoenix_MotorControl_SetStatusFramePeriod_Enhanced.vi"("periodMs"=w54, "Status Frame"=w51, "PhoenixMotorControlDevRef"=w56) -> ("PhoenixMotorControlDevRef"=w47:T20)  [unwired: 7 in, 1 out]
  n43 = call <vilib>:"CTRE_Phoenix_MotorControl_SetSensorPhase.vi"("PhaseSensor"=TRUE, "PhoenixMotorControlDevRef"=w50) -> ("PhoenixMotorControlDevRef"=w42:T20)  [unwired: 8 in, 1 out]
  n44 = call <vilib>:"CTRE_Phoenix_MotorControl_SetSensorPhase.vi"("PhaseSensor"=TRUE, "PhoenixMotorControlDevRef"=w49) -> ("PhoenixMotorControlDevRef"=w41:T20)  [unwired: 8 in, 1 out]
  n45 = call <vilib>:"CTRE_Phoenix_MotorControl_SetSensorPhase.vi"("PhaseSensor"=TRUE, "PhoenixMotorControlDevRef"=w48) -> ("PhoenixMotorControlDevRef"=w40:T20)  [unwired: 8 in, 1 out]
  n46 = call <vilib>:"CTRE_Phoenix_MotorControl_SetSensorPhase.vi"("PhaseSensor"=TRUE, "PhoenixMotorControlDevRef"=w47) -> ("PhoenixMotorControlDevRef"=w39:T20)  [unwired: 8 in, 1 out]
  n47 = disable-structure shown="Disabled" {
    frame Disabled {
      n48 = call <vilib>:"CTRE_Phoenix_TalonSRX_Open.vi"("Device Number"=u8 10) -> ("error out"=w101:errorcluster, "CAN Talon SRX Ref"=w102:T20)  [unwired: 9 in]
      n49 = call <vilib>:"CTRE_Phoenix_MotorControl_RefNumRegistrySet.vi"("error in (no error)"=w101, "refnum name"="elevatorMotor02", "PhoenixMotorControlDevRef"=w102) -> ()  [unwired: 7 in, 2 out]
    }
    frame Enabled {
    }
  }
  n50 = call <vilib>:"CTRE_Phoenix_TalonSRX_Open.vi"("Device Number"=u8 12) -> ("error out"=w85:errorcluster, "CAN Talon SRX Ref"=w86:T20)  [unwired: 9 in]
  n51 = call <vilib>:"CTRE_Phoenix_MotorControl_ConfigAllSettingsEnhanced.vi"("Enhanced Motor Controller Configurables"=w17, "PhoenixMotorControlDevRef"=w42) -> ("PhoenixMotorControlDevRef"=w38:T20)  [unwired: 8 in, 1 out]
  n52 = call <vilib>:"CTRE_Phoenix_MotorControl_ConfigAllSettingsEnhanced.vi"("Enhanced Motor Controller Configurables"=w17, "PhoenixMotorControlDevRef"=w41) -> ("PhoenixMotorControlDevRef"=w37:T20)  [unwired: 8 in, 1 out]
  n53 = call <vilib>:"CTRE_Phoenix_MotorControl_ConfigAllSettingsEnhanced.vi"("Enhanced Motor Controller Configurables"=w18, "PhoenixMotorControlDevRef"=w40) -> ("PhoenixMotorControlDevRef"=w36:T20)  [unwired: 8 in, 1 out]
  n54 = call <vilib>:"CTRE_Phoenix_MotorControl_ConfigAllSettingsEnhanced.vi"("Enhanced Motor Controller Configurables"=w18, "PhoenixMotorControlDevRef"=w39) -> ("PhoenixMotorControlDevRef"=w35:T20)  [unwired: 8 in, 1 out]
  n55 = call <vilib>:"CTRE_Phoenix_MotorControl_RefNumRegistrySet.vi"("error in (no error)"=w85, "refnum name"="elevatorMotor01", "PhoenixMotorControlDevRef"=w86) -> ()  [unwired: 7 in, 2 out]
  n56 = call-poly <vilib>:"WPI_RobotDriveOpen4Motor.vi"("Rear Left Motor Dev Ref"=w38, "Rear Right Motor Dev Ref"=w37, "Front Left Motor Dev Ref"=w36, "Front Right Motor Dev Ref"=w35) -> ("RobotDriveDevRef"=w77:T25)  [unwired: 10 in, 1 out]
  n57 = call <vilib>:"WPI_RobotDriveRefNum Registry Set.vi"("refnum name"="driveMotors", "RobotDriveDevRef"=w77) -> ()  [unwired: 8 in, 2 out]
  n58 = disable-structure shown="Disabled" {
    frame Disabled {
      w119 = cluster{"P":dbl, "I":dbl, "D":dbl, "F":dbl} {"P"=0.0, "I"=0.0, "D"=0.0, "F"=0.0}  # Back Motor PIDF Values
      w120 = cluster{"P":dbl, "I":dbl, "D":dbl, "F":dbl} {"P"=0.0, "I"=0.0, "D"=0.0, "F"=0.0}  # Front Motor PIDF Values
      w137 = T19 5696 items=["Status_1_General"=5120, "Status_2_Feedback0"=5184, "Status_3_Quadrature"=5248, "Status_4_AinTempVbat"=5312, "Status_6_Misc"=5440, "Status_7_CommStatus"=5504, "Status_8_PulseWidth"=5568, "Status_9_MotProfBuffer"=5632, "Status_10_MotionMagic"=5696, "Status_11_UartGadgeteer"=5760, "Status_12_Feedback1"=5824, "Status_13_Base_PIDF0"=5888, "Status_14_Turn_PIDF1"=5952, "Status_15_FirmwareApiStatus"=6016] ("Status Frame")
      w139 = T19 5632 items=["Status_1_General"=5120, "Status_2_Feedback0"=5184, "Status_3_Quadrature"=5248, "Status_4_AinTempVbat"=5312, "Status_6_Misc"=5440, "Status_7_CommStatus"=5504, "Status_8_PulseWidth"=5568, "Status_9_MotProfBuffer"=5632, "Status_10_MotionMagic"=5696, "Status_11_UartGadgeteer"=5760, "Status_12_Feedback1"=5824, "Status_13_Base_PIDF0"=5888, "Status_14_Turn_PIDF1"=5952, "Status_15_FirmwareApiStatus"=6016] ("Status Frame")
      w141 = 7
      w140 = 10
      w149 = 10
      w154 = 1.5
      # "Front Right"
      # "Front Left"
      # "Rear Right"
      # "Rear Left"
      n59 = call <vilib>:"CTRE_Phoenix_TalonFX_Open.vi"("Device Number"=u8 0) -> ("CAN Talon SRX Ref"=w158:T20)  [unwired: 9 in, 1 out]
      n60 = call <vilib>:"CTRE_Phoenix_TalonFX_Open.vi"("Device Number"=u8 2) -> ("CAN Talon SRX Ref"=w156:T20)  [unwired: 9 in, 1 out]
      n61 = call <vilib>:"CTRE_Phoenix_TalonFX_Open.vi"("Device Number"=u8 1) -> ("CAN Talon SRX Ref"=w157:T20)  [unwired: 9 in, 1 out]
      n62 = call <vilib>:"CTRE_Phoenix_TalonFX_Open.vi"("Device Number"=u8 3) -> ("CAN Talon SRX Ref"=w155:T20)  [unwired: 9 in, 1 out]
      n63 = call <vilib>:"CTRE_Phoenix_MotorControl_ConfigOpenLoopRamp.vi"("secondsFromNeutralToFull"=w154, "PhoenixMotorControlDevRef"=w158) -> ("PhoenixMotorControlDevRef"=w153:T20)  [unwired: 8 in, 1 out]
      n64 = call <vilib>:"CTRE_Phoenix_MotorControl_ConfigOpenLoopRamp.vi"("secondsFromNeutralToFull"=w154, "PhoenixMotorControlDevRef"=w157) -> ("PhoenixMotorControlDevRef"=w152:T20)  [unwired: 8 in, 1 out]
      n65 = call <vilib>:"CTRE_Phoenix_MotorControl_ConfigOpenLoopRamp.vi"("secondsFromNeutralToFull"=w154, "PhoenixMotorControlDevRef"=w156) -> ("PhoenixMotorControlDevRef"=w151:T20)  [unwired: 8 in, 1 out]
      n66 = call <vilib>:"CTRE_Phoenix_MotorControl_ConfigOpenLoopRamp.vi"("secondsFromNeutralToFull"=w154, "PhoenixMotorControlDevRef"=w155) -> ("PhoenixMotorControlDevRef"=w150:T20)  [unwired: 8 in, 1 out]
      n67 = Select(t="Front Motor PIDF Values", s="Tune PIDF Manually?", f=w120) -> (s? t:f=w116:cluster{"P":dbl, "I":dbl, "D":dbl, "F":dbl})
      n68 = Select(t="Back Motor PIDF Values", s="Tune PIDF Manually?", f=w119) -> (s? t:f=w115:cluster{"P":dbl, "I":dbl, "D":dbl, "F":dbl})
      n69 = call <vilib>:"CTRE_Phoenix_MotorControl_ChangeMotionControlFramePeriod.vi"("periodMs"=w149, "PhoenixMotorControlDevRef"=w153) -> ("PhoenixMotorControlDevRef"=w148:T20)  [unwired: 8 in, 1 out]
      n70 = call <vilib>:"CTRE_Phoenix_MotorControl_ChangeMotionControlFramePeriod.vi"("periodMs"=w149, "PhoenixMotorControlDevRef"=w152) -> ("PhoenixMotorControlDevRef"=w147:T20)  [unwired: 8 in, 1 out]
      n71 = call <vilib>:"CTRE_Phoenix_MotorControl_ChangeMotionControlFramePeriod.vi"("periodMs"=w149, "PhoenixMotorControlDevRef"=w151) -> ("PhoenixMotorControlDevRef"=w146:T20)  [unwired: 8 in, 1 out]
      n72 = call <vilib>:"CTRE_Phoenix_MotorControl_ChangeMotionControlFramePeriod.vi"("periodMs"=w149, "PhoenixMotorControlDevRef"=w150) -> ("PhoenixMotorControlDevRef"=w145:T20)  [unwired: 8 in, 1 out]
      n73 = Unbundle By Name(w116) -> ("P"=w114:dbl, "I"=w113:dbl, "D"=w112:dbl, "F"=w111:dbl)
      n74 = Unbundle By Name(w115) -> ("P"=w110:dbl, "I"=w109:dbl, "D"=w108:dbl, "F"=w107:dbl)
      n75 = call <vilib>:"CTRE_Phoenix_MotorControl_SetStatusFramePeriod_Enhanced.vi"("periodMs"=w141, "Status Frame"=w139, "PhoenixMotorControlDevRef"=w148) -> ("PhoenixMotorControlDevRef"=w144:T20)  [unwired: 7 in, 1 out]
      n76 = call <vilib>:"CTRE_Phoenix_MotorControl_SetStatusFramePeriod_Enhanced.vi"("periodMs"=w141, "Status Frame"=w139, "PhoenixMotorControlDevRef"=w147) -> ("PhoenixMotorControlDevRef"=w143:T20)  [unwired: 7 in, 1 out]
      n77 = call <vilib>:"CTRE_Phoenix_MotorControl_SetStatusFramePeriod_Enhanced.vi"("periodMs"=w141, "Status Frame"=w139, "PhoenixMotorControlDevRef"=w146) -> ("PhoenixMotorControlDevRef"=w138:T20)  [unwired: 7 in, 1 out]
      n78 = call <vilib>:"CTRE_Phoenix_MotorControl_SetStatusFramePeriod_Enhanced.vi"("periodMs"=w141, "Status Frame"=w139, "PhoenixMotorControlDevRef"=w145) -> ("PhoenixMotorControlDevRef"=w142:T20)  [unwired: 7 in, 1 out]
      n79 = Bundle By Name(cluster="Talon FX Configurables", "Base Configurables.slot3.P"=w110, "Base Configurables.slot3.I"=w109, "Base Configurables.slot3.D"=w108, "Base Configurables.slot3.F"=w107) -> (w104:T1)
      n80 = Bundle By Name(cluster="Talon FX Configurables", "Base Configurables.slot2.P"=w114, "Base Configurables.slot2.I"=w113, "Base Configurables.slot2.D"=w112, "Base Configurables.slot2.F"=w111) -> (w105:T1)
      n81 = call <vilib>:"CTRE_Phoenix_MotorControl_SetStatusFramePeriod_Enhanced.vi"("periodMs"=w140, "Status Frame"=w137, "PhoenixMotorControlDevRef"=w144) -> ("PhoenixMotorControlDevRef"=w136:T20)  [unwired: 7 in, 1 out]
      n82 = call <vilib>:"CTRE_Phoenix_MotorControl_SetStatusFramePeriod_Enhanced.vi"("periodMs"=w140, "Status Frame"=w137, "PhoenixMotorControlDevRef"=w143) -> ("PhoenixMotorControlDevRef"=w135:T20)  [unwired: 7 in, 1 out]
      n83 = call <vilib>:"CTRE_Phoenix_MotorControl_SetStatusFramePeriod_Enhanced.vi"("periodMs"=w140, "Status Frame"=w137, "PhoenixMotorControlDevRef"=w138) -> ("PhoenixMotorControlDevRef"=w134:T20)  [unwired: 7 in, 1 out]
      n84 = call <vilib>:"CTRE_Phoenix_MotorControl_SetStatusFramePeriod_Enhanced.vi"("periodMs"=w140, "Status Frame"=w137, "PhoenixMotorControlDevRef"=w142) -> ("PhoenixMotorControlDevRef"=w133:T20)  [unwired: 7 in, 1 out]
      n85 = call <vilib>:"CTRE_Phoenix_MotorControl_SetSensorPhase.vi"("PhaseSensor"=TRUE, "PhoenixMotorControlDevRef"=w136) -> ("PhoenixMotorControlDevRef"=w128:T20)  [unwired: 8 in, 1 out]
      n86 = call <vilib>:"CTRE_Phoenix_MotorControl_SetSensorPhase.vi"("PhaseSensor"=FALSE, "PhoenixMotorControlDevRef"=w135) -> ("PhoenixMotorControlDevRef"=w127:T20)  [unwired: 8 in, 1 out]
      n87 = call <vilib>:"CTRE_Phoenix_MotorControl_SetSensorPhase.vi"("PhaseSensor"=TRUE, "PhoenixMotorControlDevRef"=w134) -> ("PhoenixMotorControlDevRef"=w126:T20)  [unwired: 8 in, 1 out]
      n88 = call <vilib>:"CTRE_Phoenix_MotorControl_SetSensorPhase.vi"("PhaseSensor"=FALSE, "PhoenixMotorControlDevRef"=w133) -> ("PhoenixMotorControlDevRef"=w125:T20)  [unwired: 8 in, 1 out]
      n89 = call <vilib>:"CTRE_Phoenix_MotorControl_ConfigAllSettings_TalonFX.vi"("Talon FX Configurables"=w104, "PhoenixMotorControlDevRef"=w128) -> ("PhoenixMotorControlDevRef"=w124:T20)  [unwired: 8 in, 1 out]
      n90 = call <vilib>:"CTRE_Phoenix_MotorControl_ConfigAllSettings_TalonFX.vi"("Talon FX Configurables"=w104, "PhoenixMotorControlDevRef"=w127) -> ("PhoenixMotorControlDevRef"=w123:T20)  [unwired: 8 in, 1 out]
      n91 = call <vilib>:"CTRE_Phoenix_MotorControl_ConfigAllSettings_TalonFX.vi"("Talon FX Configurables"=w105, "PhoenixMotorControlDevRef"=w126) -> ("PhoenixMotorControlDevRef"=w122:T20)  [unwired: 8 in, 1 out]
      n92 = call <vilib>:"CTRE_Phoenix_MotorControl_ConfigAllSettings_TalonFX.vi"("Talon FX Configurables"=w105, "PhoenixMotorControlDevRef"=w125) -> ("PhoenixMotorControlDevRef"=w121:T20)  [unwired: 8 in, 1 out]
      n93 = call-poly <vilib>:"WPI_RobotDriveOpen4Motor.vi"("Rear Left Motor Dev Ref"=w124, "Rear Right Motor Dev Ref"=w123, "Front Left Motor Dev Ref"=w122, "Front Right Motor Dev Ref"=w121) -> ("RobotDriveDevRef"=w163:T25)  [unwired: 10 in, 1 out]
      n94 = call <vilib>:"WPI_RobotDriveRefNum Registry Set.vi"("refnum name"="driveMotors", "RobotDriveDevRef"=w163) -> ()  [unwired: 8 in, 2 out]
    }
    frame Enabled {
    }
  }
